vi "is_a_digit.vi"(10 "String":string) -> (2 "is a digit":bool)   [LabVIEW 2013]
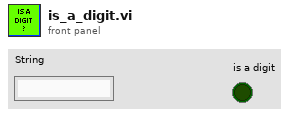
[diagram p1: front panel]
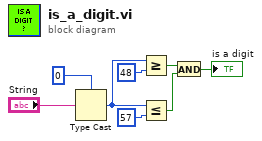
[diagram p0: block diagram]
diagram:
  n1 = Type Cast(type=u8 0, x="String") -> (*(type *) &x=w2:u8)
  n2 = Greater Or Equal?(x=w2, y=u8 48) -> (x >= y?=w4:bool)
  n3 = Less Or Equal?(x=w2, y=u8 57) -> (x <= y?=w3:bool)
  n4 = And(x=w4, y=w3) -> (x .and. y?=→"is a digit":bool)
